vi "Execute.vi"(8 "Error In":errorcluster, 9 "Workspace":T1, 10 "Control In":T2={"I-O.lvclass"=refnum, "Motion.lvclass"=refnum, "Dispenser.lvclass"=refnum}, 11 "CAD Dispense2 in":refnum<class "CAD Dispense2.lvclass">) -> (0 "Error Out":errorcluster, 2 "Control Out":T2, 3 "CAD Dispense2 in 2":refnum<class "CAD Dispense2.lvclass">)   [LabVIEW 2016, in "CAD Dispense2.lvclass"]
uses:
  CAD Dispense2.lvclass
  D:/UCSB-Gantry 0418/V5/Classes/Routine/Dispense/Dispense.lvclass
  Controller/Controllers.ctl
  Controller/I-O/I-O.lvclass
  Controller/Motion/A3200/A3200.lvclass
  Controller/Dispenser/Dispenser.lvclass
  Controller/Motion/Motion.lvclass
  Workspace/Workspace.ctl
  Dispense.lvclass/Dispense.ctl
  Read Timing Data (Go Down and Dispense).vi
  Read Timing Path.vi
  Read Time.vi
  Read Pattern Coordinates.vi
  Read Tip Height.vi
  Dispense.lvclass
  Controller/Controller.lvclass
  Workspace/Fixture.lvclass
panel:
  out "XYZTheta 2":dbl[](array[numeric])
  out "XYZTheta":dbl[](array[numeric])
  out "Pattern Coordinates":dbl[][](array[numeric])
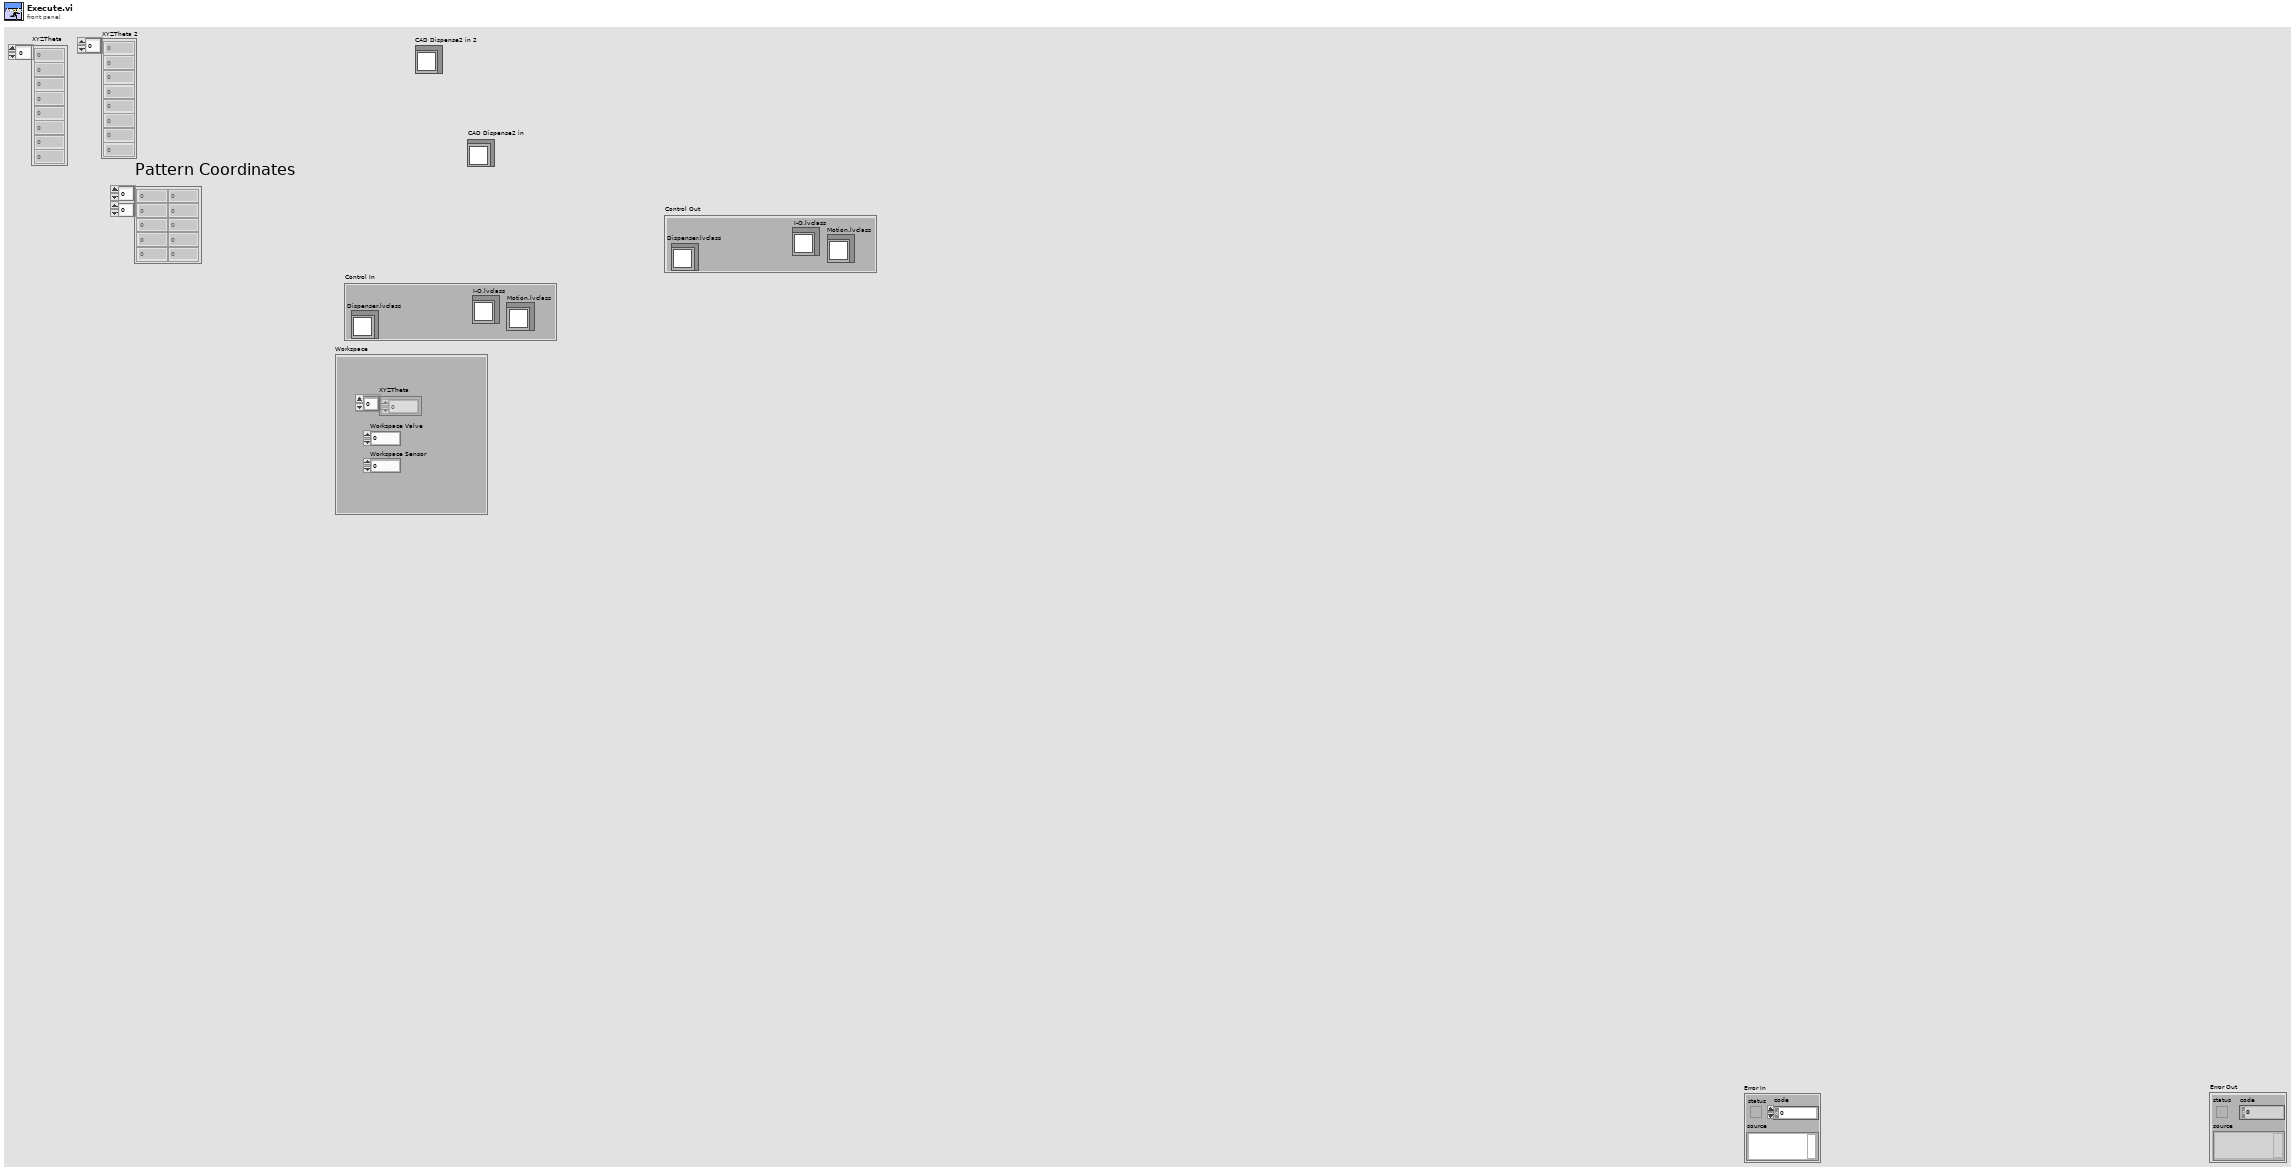
[diagram p1: front panel]
types:
  T1 = typedef "Fixture.lvclass/Workspace.ctl" = cluster{"XYZTheta":dbl[], "Workspace Valve":i32, "Workspace Sensor":i32}
  T2 = typedef "Controller.lvclass/Controllers.ctl" = cluster{"I-O.lvclass":refnum<class "I-O.lvclass">, "Motion.lvclass":refnum<class "Motion.lvclass">, "Dispenser.lvclass":refnum<class "Dispenser.lvclass">}
  T3 = cluster{"Time to Go Down":dbl, "Time to Dispense":dbl}[]
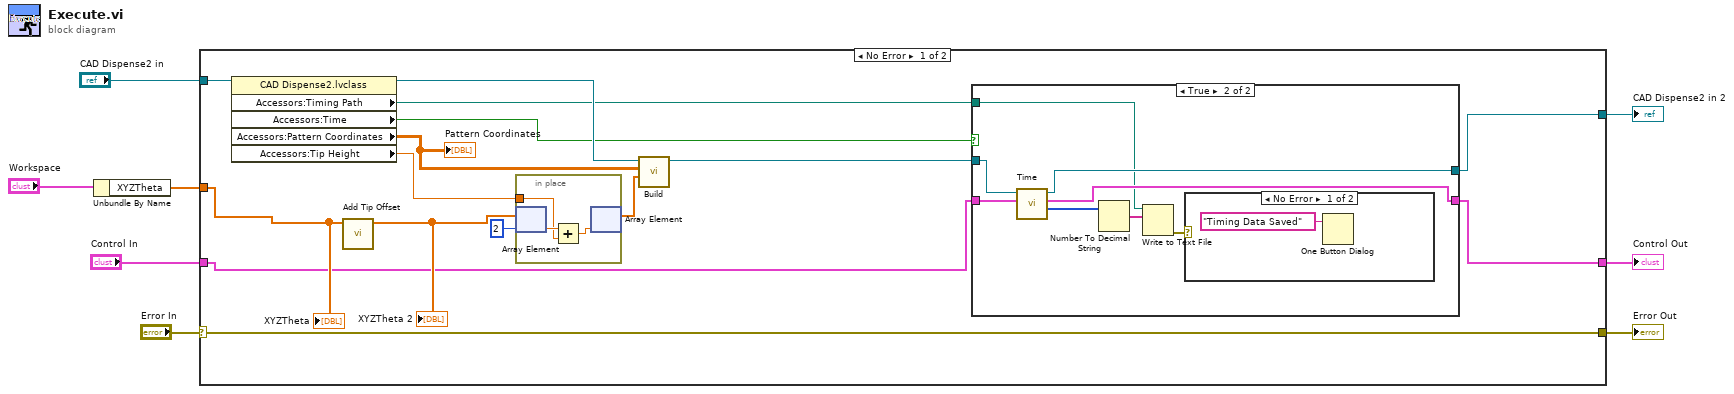
[diagram p0: block diagram]
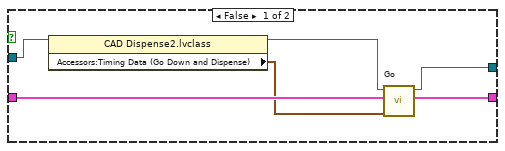
[diagram p2: hidden frame]
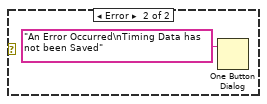
[diagram p3: hidden frame]
diagram:
  n1 = Unbundle By Name("Workspace") -> ("XYZTheta"=w2:dbl[])
  n2 = case shown="No Error" "Error In" {
    selector: "Error In" -> [w23 w45]
    tunnel: [w23 w45] -> w7
    tunnel: "CAD Dispense2 in" -> [w15 w44]
    tunnel: [w16 w44] -> w6
    tunnel: "Control In" -> [w18 w43]
    tunnel: [w17 w43] -> w4
    tunnel: w2 -> [w19 _]
    frame No Error {
      n3 = property class="CAD Dispense2.lvclass"(reference=w15) -> (reference out=w14:refnum<class "CAD Dispense2.lvclass">, "Accessors:Timing Path"=w9:path, "Accessors:Time"=w10:bool, "Accessors:Pattern Coordinates"=w13:dbl[][], "Accessors:Tip Height"=w12:dbl)  [unwired: 1 in, 1 out]
      "Pattern Coordinates" <- w13
      n4 = call "Add Tip Offset.vi"("XYZTheta"=w19) -> ("XYZTheta"=w20:dbl[])  [unwired: 10 in]
      "XYZTheta 2" <- w20
      n5 = in-place {
        in-place-border: w12 -> [w40]
        n6 = in-place-array #1(w20, 2) -> (w42:dbl)
        n7 = Add(x=w42, y=w40) -> (x+y=w41:dbl)
        n8 = in-place-array #1(w41) -> (w21:dbl[])  [unwired: 1 out]
      }
      n9 = call-dynamic "Build.vi"("XYZTheta"=w21, "Pattern Coordinates"=w13, "CAD Dispense2 in"=w14) -> ("CAD Dispense2 out"=w11:refnum<class "CAD Dispense2.lvclass">)  [unwired: 7 in, 1 out]
      n10 = case shown="True" w10 {
        tunnel: w11 -> [w25 w32]
        tunnel: w18 -> [w28 w34]
        tunnel: [w29 w33] -> w17
        tunnel: [w27 w31] -> w16
        tunnel: w9 -> [_ w30]
        frame False {
          n11 = property class="CAD Dispense2.lvclass"(reference=w25) -> (reference out=w26:refnum<class "CAD Dispense2.lvclass">, "Accessors:Timing Data (Go Down and Dispense)"=w24:T3)  [unwired: 1 in, 1 out]
          n12 = call-dynamic "Go.vi"("Timing Data (Go Down and Dispense)"=w24, "Control In"=w28, "CAD Dispense2 in"=w26) -> ("Control Out"=w29:T2, "CAD Dispense2 Out"=w27:refnum<class "CAD Dispense2.lvclass">)  [unwired: 7 in]
        }
        frame True {
          n13 = call-dynamic "Time.vi"("Control In"=w34, "CAD Dispense2 in"=w32) -> ("Timing Data"=w35:i32[], "Control Out"=w33:T2, "CAD Dispense2 out"=w31:refnum<class "CAD Dispense2.lvclass">)  [unwired: 6 in, 1 out]
          n14 = Number To Decimal String(number=w35) -> (decimal integer string=w36:string[])  [unwired: 1 in]
          n15 = Write to Text File(file (use dialog)=w30, text=w36) -> (error out=w37:errorcluster)  [unwired: 2 in, 2 out]
          n16 = case shown="No Error" w37 {
            frame No Error {
              n17 = One Button Dialog(message="Timing Data Saved") -> ()  [unwired: 1 in, 1 out]
            }
            frame Error {
              n18 = One Button Dialog(message="An Error Occurred\nTiming Data has not been Saved") -> ()  [unwired: 1 in, 1 out]
            }
          }
        }
      }
      "XYZTheta" <- w19
    }
    frame Error {
    }
  }
  "Control Out" <- w4
  "Error Out" <- w7
  "CAD Dispense2 in 2" <- w6
